vi "csm_lumikki_instron_init.vi"   [LabVIEW 2009]
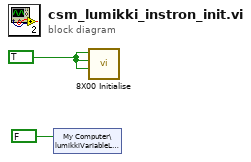
[diagram p0: block diagram]
diagram:
  w2 = TRUE ("Reset?")
  n1 = shared-variable "My Computer\\lumikkiVariableList.lvlib\\busy"(FALSE ("busy")) -> ()  [unwired: 1 in, 1 out]
  n2 = call "8X00 Initialise.vi"("Reset?"=w2, "Create DVM? (T)"=w2, "Create Console? (T)"=w2) -> ()  [unwired: 1 in, 4 out]
